vi "SPI Engine 128-bit.vi"(8 "error in":errorcluster, 10 "SPI Read Data":T4, 11 "SPI Engine Resources":T3={"To SPI Engine Data FIFO"="DLU To SPI Engine Data FIFO", "From SPI Engine Data FIFO"="SPI Engine to DLU Data FIFO", "Data to SPI Engine Cache Register"="Data to SPI Engine (Cache)", "SPI Transaction Settings Cache Register"="SPI PHY Settings to SPI Engine (Cache)"}) -> (0 "error out":errorcluster, 1 "Chip Select":u8, 2 "SPI Write Data":T5, 3 "SPI Engine Resources":T3={"To SPI Engine Data FIFO"="DLU To SPI Engine Data FIFO", "From SPI Engine Data FIFO"="SPI Engine to DLU Data FIFO", "Data to SPI Engine Cache Register"="Data to SPI Engine (Cache)", "SPI Transaction Settings Cache Register"="SPI PHY Settings to SPI Engine (Cache)"})   [LabVIEW 2015, in "SPI API.lvlib"]
doc: "This VI is the actual SPI Engine. It handles the SPI communication to the SPI bus."
uses:
  SPI API.lvlib
  <userlib>/_NI SPI IP/FPGA/Controllers/Public/Spi Master Outputs.ctl
  <userlib>/_NI SPI IP/FPGA/Controllers/Public/Spi Master Inputs.ctl
  Controls/SPI Engine Resources 128-bit.ctl
  Controls/SPI API Response Data 128-bit.ctl
  Controls/SPI API Data 128-bit.ctl
  Get SPI Engine Commands 128-bit.vi
  SPI Engine Core 128-bit.vi
  Send SPI Engine Response 128-bit.vi
  <userlib>/_NI SPI IP/FPGA/Controllers/NI SPI IP FPGA.lvlib
panel:
  out "Response Data":T1
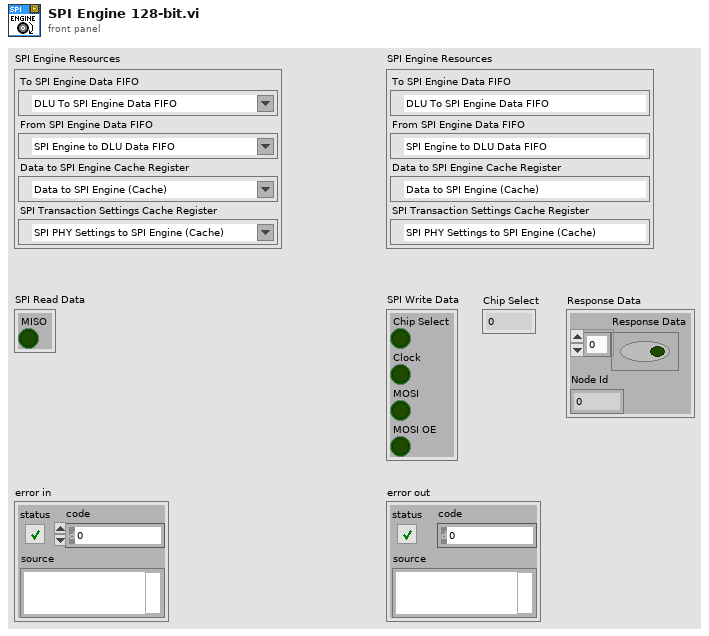
[diagram p1: front panel]
types:
  T1 = typedef "SPI API.lvlib/SPI API Response Data 128-bit.ctl" = cluster{"Response Data":T2, "Node Id":u16}
  T2 = typedef "SPI API.lvlib/SPI API Data 128-bit.ctl" = bool[]
  T3 = typedef "SPI API.lvlib/SPI Engine Resources 128-bit.ctl" = cluster{"To SPI Engine Data FIFO":refnum<k21>, "From SPI Engine Data FIFO":refnum<k21>, "Data to SPI Engine Cache Register":refnum<k21>, "SPI Transaction Settings Cache Register":refnum<k21>}
  T4 = typedef "NI SPI IP FPGA.lvlib/Spi Master Inputs.ctl" = cluster{"MISO":bool}
  T5 = typedef "NI SPI IP FPGA.lvlib/Spi Master Outputs.ctl" = cluster{"Chip Select":bool, "Clock":bool, "MOSI":bool, "MOSI OE":bool}
  T6 = typedef "SPI API.lvlib/SPI API Transaction Packet 128-bit.ctl" = cluster{"Start Strobe":bool, "SPI Data":T2, "SPI Settings":T7}
  T7 = typedef "SPI API.lvlib/SPI Transaction Settings.ctl" = cluster{"Chip Select ID":u8, "SPI Physical Settings":T8}
  T8 = typedef "NI SPI IP FPGA.lvlib/Transfer Settings.ctl" = cluster{"Divide Value":u8, "Transfer Length (bits)":u8, "CS Asserted Polarity":bool, "Clock Polarity (CPOL)":bool, "Clock Phase (CPHA)":bool, "Lengthen MISO Setup":bool, "Direction Change Bit":u8, "MOSI Starts as Output":bool, "Tristatable MOSI":bool}
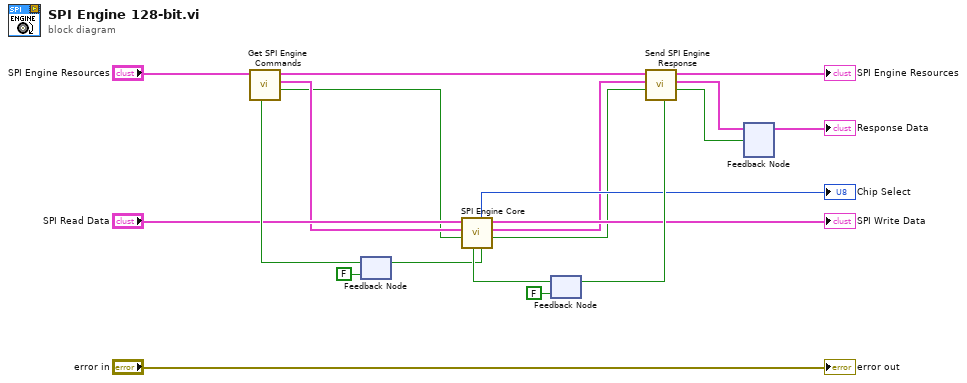
[diagram p0: block diagram]
diagram:
  n1 = feedback #1(FALSE ("ready for input")) -> (w16:bool)
  n2 = call-poly "Get SPI Engine Commands.vi"("Ready for Output"=w16, "SPI Engine Resources"="SPI Engine Resources") -> ("Output Valid"=w7:bool, "SPI Transaction Packet"=w8:T6, "SPI Engine Resources"=w15:T3)  [unwired: 5 in, 2 out]
  n3 = feedback #2(FALSE ("Ready for Input")) -> (w6:bool)
  n4 = call-poly "SPI Engine Core.vi"("Ready for Output"=w6, "Input Valid"=w7, "SPI Information In"=w8, "SPI DIO Input"="SPI Read Data") -> ("Output Valid"=w1:bool, "SPI Output Data"=w2:T1, "SPI DIO Output"=→"SPI Write Data":T5, "Ready For Input"=w5:bool, "Chip Select ID"=→"Chip Select":u8)  [unwired: 3 in]
  n5 = feedback-in #1(w5) -> ()
  n6 = call-poly "Send SPI Engine Response.vi"("Input Valid"=w1, "Response Data"=w2, "SPI Engine Resources"=w15) -> ("New Data Sent?"=w11:bool, "Response Data"=w12:T1, "SPI Engine Resources"=→"SPI Engine Resources":T3, "Ready for Input"=w13:bool)  [unwired: 4 in, 1 out]
  n7 = feedback-in #2(w13) -> ()
  n8 = feedback-in #3(w12, w11) -> ()
  n9 = feedback #3() -> (→"Response Data":T1)  [unwired: 1 in]
  "error out" <- "error in"
